vi "Test Outer Loop.vi"   [LabVIEW 2013]
uses:
  classes/Test/Test.lvclass
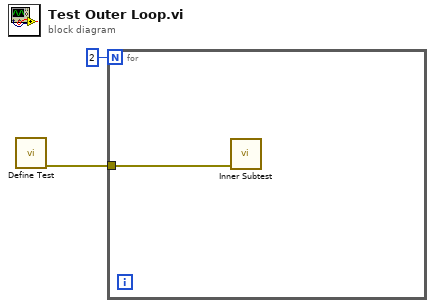
[diagram p0: block diagram]
diagram:
  n1 = call "Define Test.vi"() -> ("error out"=w1:errorcluster)  [unwired: 11 in]
  n2 = for {
    N: 2 -> [_]
    tunnel: w1 -> [w3]
    n3 = call "Inner Subtest.vi"("error in (no error)"=w3) -> ()  [unwired: 10 in, 1 out]
  }
